vi "classification.vi"() -> ()   [LabVIEW 2018]
panel:
  out "Gem Classification":string[][](array[string])
  out "Mean Classification":string[][](array[string])
  # "Add colour to the array background (if possible) perhaps using Create->Property Node or Invoke Node....\n-combine cal safety and comfort into one"
  # "GEM"
  # "MEAN"
  # "Autumn"
  # "Winter"
  # "Annual"
  # "Spring"
  # "Summer"
  # "Autumn"
  # "Winter"
  # "Annual"
  # "Spring"
  # "Summer"
  # "Probe Number"
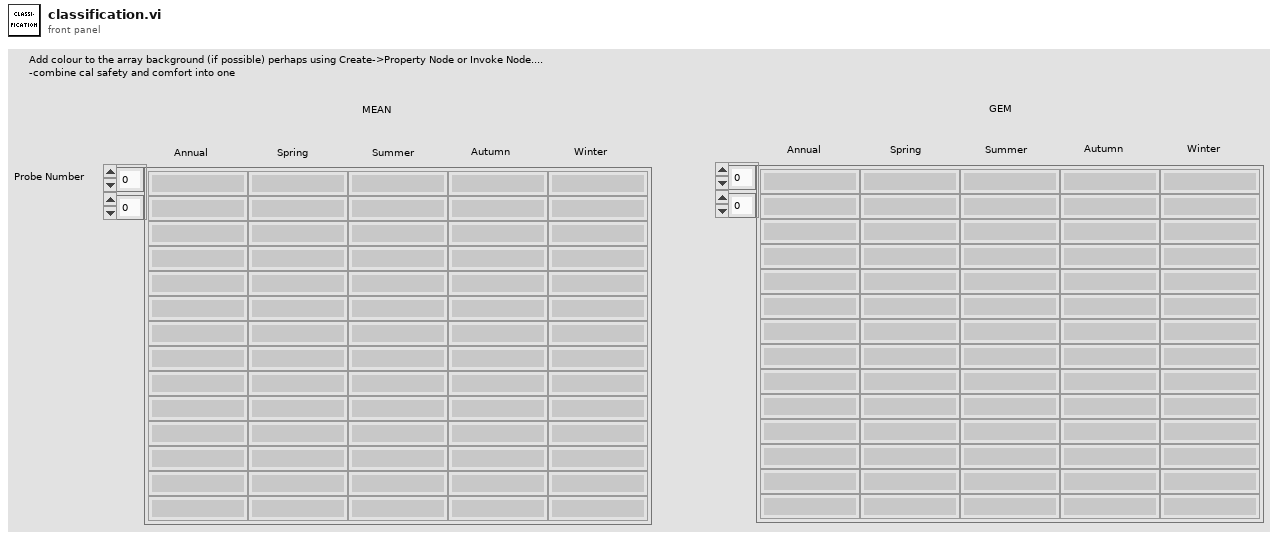
[diagram p1: front panel]
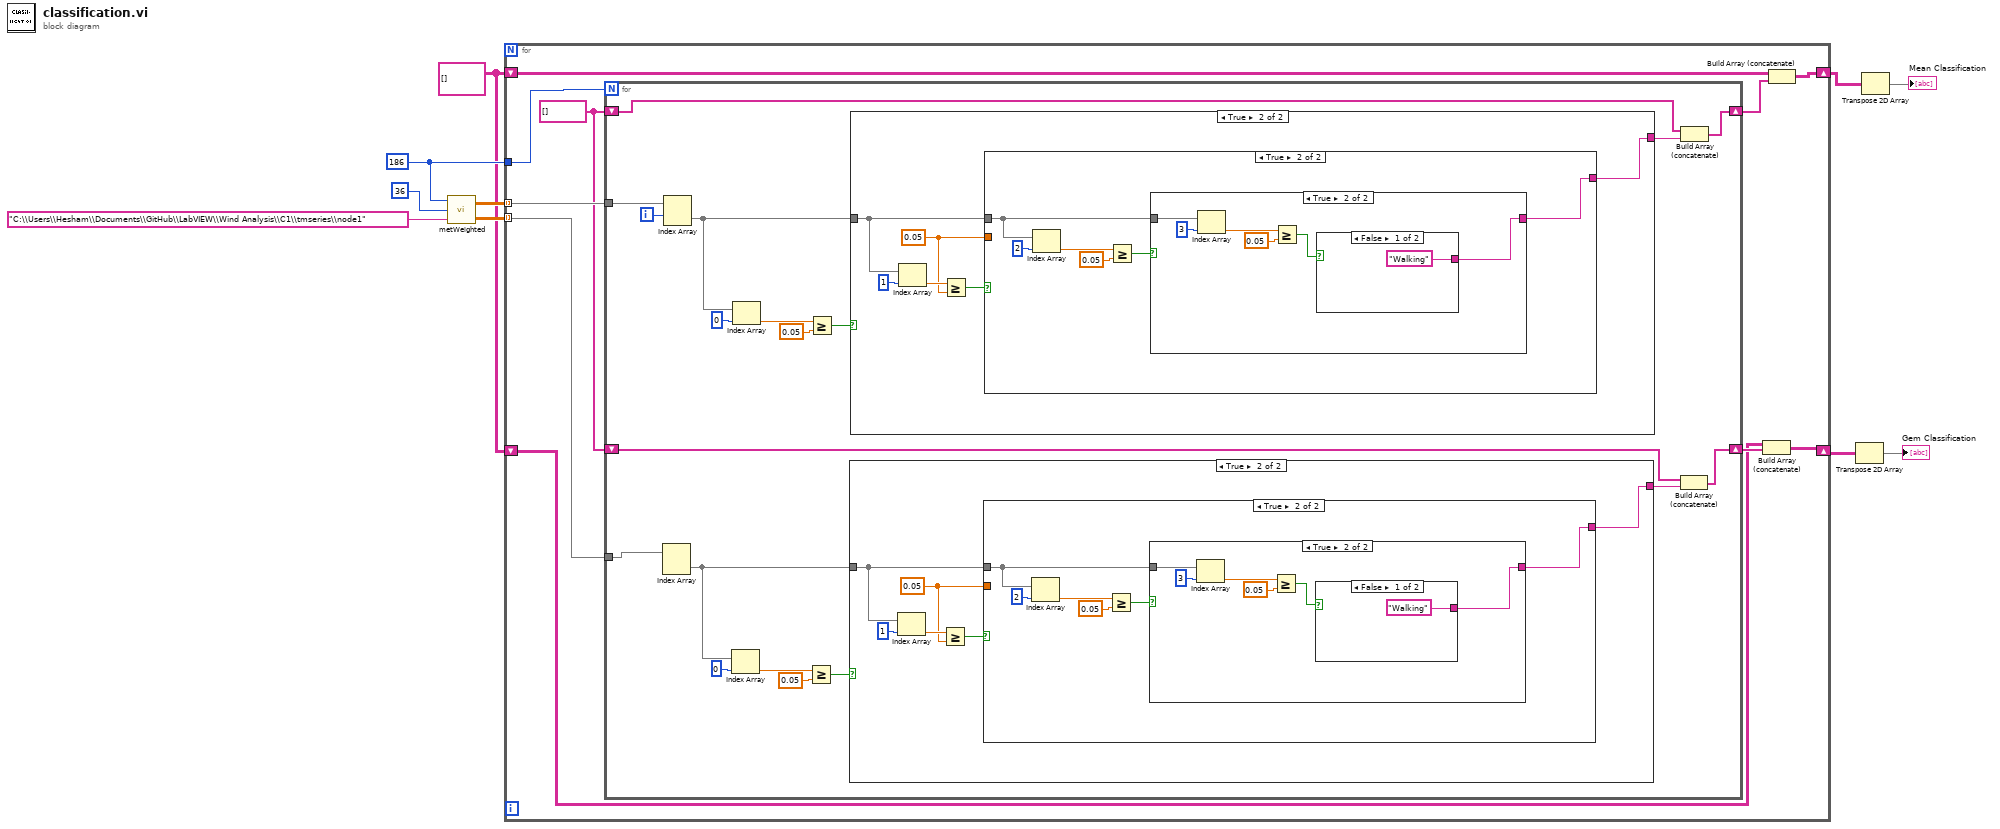
[diagram p0: block diagram]
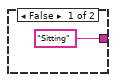
[diagram p2: hidden frame]
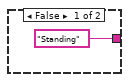
[diagram p3: hidden frame]
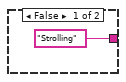
[diagram p4: hidden frame]
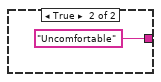
[diagram p5: hidden frame]
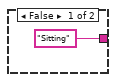
[diagram p6: hidden frame]
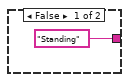
[diagram p7: hidden frame]
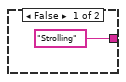
[diagram p8: hidden frame]
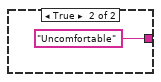
[diagram p9: hidden frame]
diagram:
  w1 = string[][] []
  w7 = 186 ("Number of Probes")
  n1 = call "metWeighted.vi"("VSERTIM Path"="C:\\Users\\Hesham\\Documents\\GitHub\\LabVIEW\\Wind Analysis\\C1\\tmseries\\node1", "Number of Angles"=36, "Number of Probes"=w7) -> ("tgemEx"=w4:dbl[][][], "tmeanEx"=w10:dbl[][][])
  n2 = for {
    tunnel: w10 -> [w20] mode=indexing
    tunnel: w7 -> [w19]
    shift-right: [w17] -> w9
    shift-left: w1 -> [w16]
    tunnel: w4 -> [w14] mode=indexing
    shift-right: [w12] -> w2
    shift-left: w1 -> [w11]
    w15 = string[] []
    n3 = for {
      N: w19 -> [_]
      tunnel: w20 -> [w39]
      shift-right: [w31] -> w18
      shift-left: w15 -> [w30]
      shift-right: [w21] -> w13
      shift-left: w15 -> [w23]
      tunnel: w14 -> [w22]
      i -> [w38]
      n4 = Index Array(array=w22) -> (element=w28:dbl[])  [unwired: 2 in]
      n5 = Index Array(array=w39, index (row)=w38) -> (element=w33:dbl[])  [unwired: 1 in]
      n6 = Index Array(array=w28, index=0) -> (element=w27:dbl)
      n7 = Index Array(array=w33, index=0) -> (element=w34:dbl)
      n8 = Greater Or Equal?(x=w27, y=0.05) -> (x >= y?=w25:bool)
      n9 = Greater Or Equal?(x=w34, y=0.05) -> (x >= y?=w36:bool)
      n10 = case shown="True" w25 {
        tunnel: w28 -> [_ w44]
        tunnel: ["Sitting" w43] -> w29
        frame False {
        }
        frame True {
          w41 = 0.05 ("y")
          n11 = Index Array(array=w44, index=1) -> (element=w42:dbl)
          n12 = Greater Or Equal?(x=w42, y=w41) -> (x >= y?=w45:bool)
          n13 = case shown="True" w45 {
            tunnel: w44 -> [_ w49]
            tunnel: ["Standing" w48] -> w43
            tunnel: w41 -> [_ _]
            frame False {
            }
            frame True {
              n14 = Index Array(array=w49, index=2) -> (element=w51:dbl)
              n15 = Greater Or Equal?(x=w51, y=0.05) -> (x >= y?=w50:bool)
              n16 = case shown="True" w50 {
                tunnel: w49 -> [_ w56]
                tunnel: ["Strolling" w55] -> w48
                frame False {
                }
                frame True {
                  n17 = Index Array(array=w56, index=3) -> (element=w58:dbl)
                  n18 = Greater Or Equal?(x=w58, y=0.05) -> (x >= y?=w57:bool)
                  n19 = case shown="False" w57 {
                    tunnel: ["Walking" "Uncomfortable"] -> w55
                    frame False {
                    }
                    frame True {
                    }
                  }
                }
              }
            }
          }
        }
      }
      n20 = case shown="True" w36 {
        tunnel: w33 -> [_ w67]
        tunnel: ["Sitting" w66] -> w32
        frame False {
        }
        frame True {
          w64 = 0.05 ("y")
          n21 = Index Array(array=w67, index=1) -> (element=w65:dbl)
          n22 = Greater Or Equal?(x=w65, y=w64) -> (x >= y?=w68:bool)
          n23 = case shown="True" w68 {
            tunnel: w67 -> [_ w72]
            tunnel: ["Standing" w71] -> w66
            tunnel: w64 -> [_ _]
            frame False {
            }
            frame True {
              n24 = Index Array(array=w72, index=2) -> (element=w74:dbl)
              n25 = Greater Or Equal?(x=w74, y=0.05) -> (x >= y?=w73:bool)
              n26 = case shown="True" w73 {
                tunnel: w72 -> [_ w79]
                tunnel: ["Strolling" w78] -> w71
                frame False {
                }
                frame True {
                  n27 = Index Array(array=w79, index=3) -> (element=w81:dbl)
                  n28 = Greater Or Equal?(x=w81, y=0.05) -> (x >= y?=w80:bool)
                  n29 = case shown="False" w80 {
                    tunnel: ["Walking" "Uncomfortable"] -> w78
                    frame False {
                    }
                    frame True {
                    }
                  }
                }
              }
            }
          }
        }
      }
      n30 = Build Array (concatenate)(w23, w29) -> (w21:string[])
      n31 = Build Array (concatenate)(w30, w32) -> (w31:string[])
    }
    n32 = Build Array (concatenate)(w11, w13) -> (w12:string[][])
    n33 = Build Array (concatenate)(w16, w18) -> (w17:string[][])
  }
  n34 = Transpose 2D Array(2D array=w2) -> (transposed array=→"Gem Classification":string[][])
  n35 = Transpose 2D Array(2D array=w9) -> (transposed array=→"Mean Classification":string[][])
